vi "TCP-VISA.vi"() -> ()   [LabVIEW 2016]
panel:
  out "Waveform Chart":dbl(graph)
  out "field value":dbl
  in  "VISA resource name":refnum<visa-resource-name>="TCPIP0::192.168.1.160::966::SOCKET"
  in  "byte count":u32=15
  out "Iteration":i32
  in  "Loop multiple (ms)":u32=500
  in  "stop":bool
  out "read buffer":string
  out "error out":errorcluster
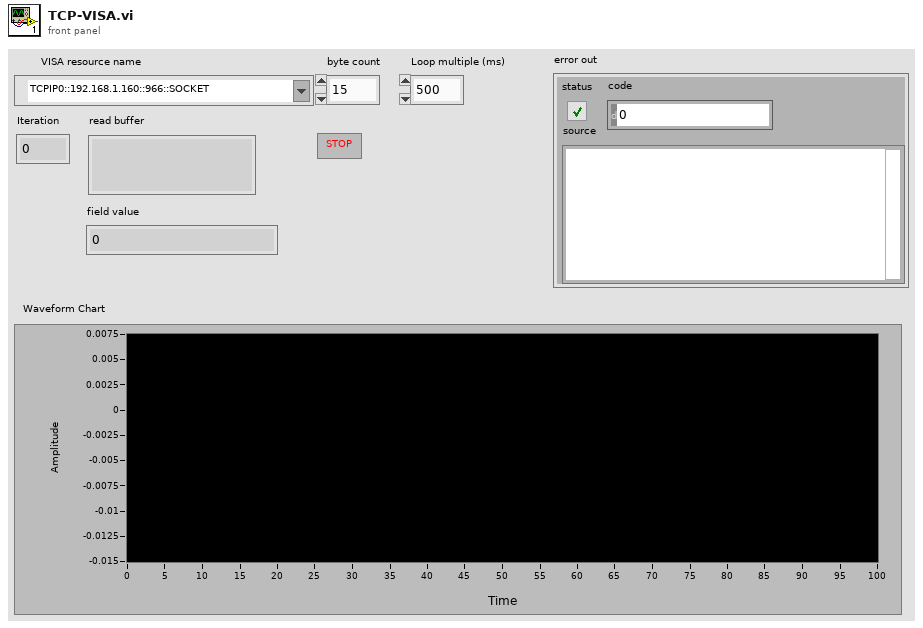
[diagram p1: front panel]
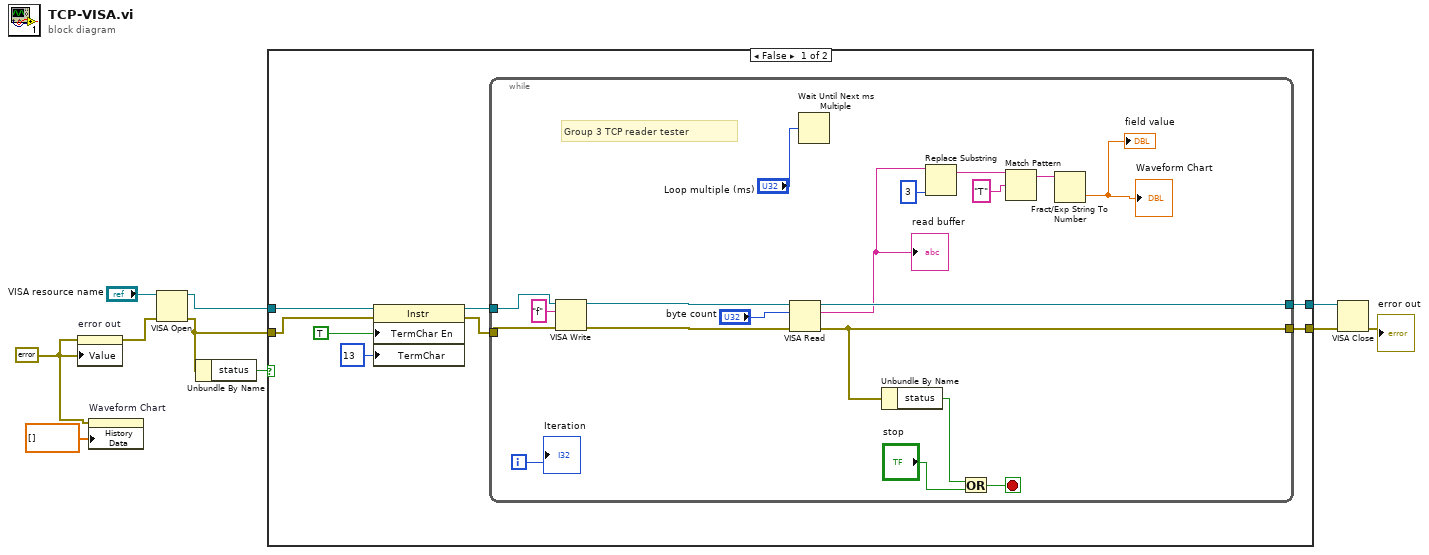
[diagram p0: block diagram]
diagram:
  w1 = errorcluster {"status"=FALSE, "code"=0, "source"=""} ("error in (no error)")
  n1 = property on="error out" class="Clust (strict)"(error in=w1, "Value"=w1) -> (error out=w4:errorcluster)  [unwired: 1 in, 1 out]
  n2 = property on="Waveform Chart" class="WFChart (strict)"(error in=w1, "History Data"=dbl[] []) -> ()  [unwired: 1 in, 2 out]
  n3 = VISA Open(error in (no error)=w4, VISA resource name="VISA resource name") -> (VISA resource name=w10:refnum<visa-resource-name>, error out=w6:errorcluster)  [unwired: 3 in]
  n4 = Unbundle By Name(w6) -> ("status"=w5:bool)
  n5 = case shown="False" w5 {
    tunnel: w10 -> [w15 w38]
    tunnel: [w18 w38] -> w9
    tunnel: w6 -> [w16 w39]
    tunnel: [w17 w39] -> w8
    frame False {
      n6 = property class="Instr"(reference=w15, error in=w16, "TermChar En"=TRUE ("Message Based Settings:Termination Character Enable"), "TermChar"=u8 13 ("Message Based Settings:Termination Character")) -> (reference out=w14:refnum<visa-resource-name>, error out=w13:errorcluster)
      n7 = while {
        tunnel: w14 -> [w26]
        tunnel: [w35] -> w18
        tunnel: w13 -> [w34]
        tunnel: [w31] -> w17
        i -> [w27]
        stop <- w29 stop-if-true
        # "Group 3 TCP reader tester"
        n8 = VISA Write(VISA resource name=w26, write buffer="f" ("data in"), error in (no error)=w34) -> (VISA resource name out=w36:refnum<visa-resource-name>, error out=w33:errorcluster)  [unwired: 1 out]
        n9 = VISA Read(VISA resource name=w36, byte count="byte count", error in (no error)=w33) -> (VISA resource name out=w35:refnum<visa-resource-name>, read buffer=w20:string, error out=w31:errorcluster)  [unwired: 1 out]
        "read buffer" <- w20
        n10 = Wait Until Next ms Multiple(millisecond multiple="Loop multiple (ms)") -> ()  [unwired: 1 out]
        n11 = Unbundle By Name(w31) -> ("status"=w30:bool)
        n12 = Replace Substring(2:3 ("length (len. of substring)"), 5:w20) -> (1:w22:string)  [unwired: 2 in, 1 out]
        n13 = Or(x=w30, y="stop") -> (x .or. y?=w29:bool)
        n14 = Match Pattern(string=w22, regular expression="T") -> (before substring=w23:string)  [unwired: 1 in, 3 out]
        n15 = Fract/Exp String To Number(string=w23) -> (number=→"field value" →"Waveform Chart":dbl)  [unwired: 3 in, 1 out]
        "Iteration" <- w27
      }
    }
    frame True {
    }
  }
  n16 = VISA Close(VISA resource name=w9, error in (no error)=w8) -> (error out=→"error out":errorcluster)
